vi "Get Column Data.vi"(8 "error in (no error)":errorcluster, 9 "Column Conditions[] (Optional)":T1[](array[typedef]), 10 "Header":string, 11 "SLL Table in":refnum<class "SLL Table.lvclass">) -> (0 "error out":errorcluster, 1 "Found?":bool, 2 "Data[]":string[](array[string]), 3 "SLL Table out":refnum<class "SLL Table.lvclass">)   [LabVIEW 2014, in "SLL Table.lvclass"]
doc: "For the specified column, returns the corresponding column data."
uses:
  SLL Table.lvclass
  _Typedefs/ColumnConditionCluster.ctl
  SLL String/_SubVIs/Search 1D String Array First Match.vi
  SLL String/SLL String.lvlib
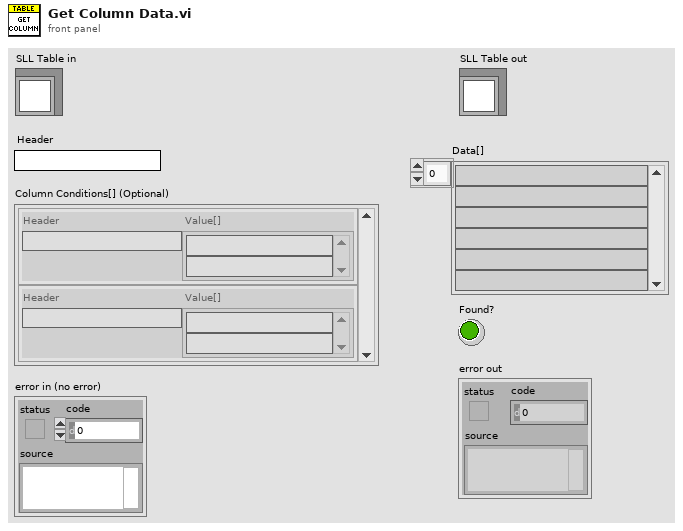
[diagram p1: front panel]
types:
  T1 = typedef "ColumnConditionCluster.ctl" = cluster{"Header":string, "Value[]":string[]}
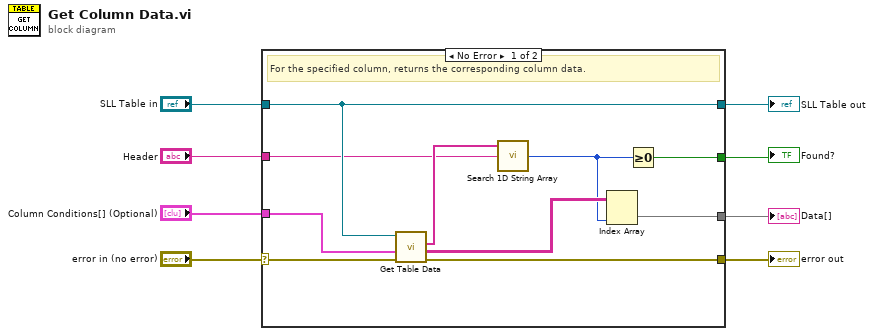
[diagram p0: block diagram]
diagram:
  n1 = case shown="No Error" "error in (no error)" {
    selector: "error in (no error)" -> [w18 w20]
    tunnel: [w17 w20] -> w7
    tunnel: [w16 w19] -> w5
    tunnel: "SLL Table in" -> [w16 w19]
    tunnel: "Header" -> [w13 _]
    tunnel: [w11 _] -> w3
    tunnel: [w9 _] -> w2
    tunnel: "Column Conditions[] (Optional)" -> [w15 _]
    frame No Error {
      # "For the specified column, returns the corresponding column data."
      n2 = call "Get Table Data.vi"("error in (no error)"=w18, "Column Conditions[] (Optional)"=w15, "SLL Table in"=w16) -> ("error out"=w17:errorcluster, "2D Data Out[][]"=w12:string[][], "Headers Out[]"=w14:string[])  [unwired: 5 in, 1 out]
      n3 = call-poly "Search 1D String Array.vi"("Element"=w13, "1D String Array"=w14) -> ("Index"=w10:i32)  [unwired: 1 in]
      n4 = Index Array(array=w12, index (col)=w10) -> (element=w11:string[])  [unwired: 1 in]
      n5 = Greater Or Equal To 0?(x=w10) -> (x >= 0?=w9:bool)
    }
    frame Error {
    }
  }
  "error out" <- w7
  "SLL Table out" <- w5
  "Data[]" <- w3
  "Found?" <- w2
